vi "Delete by Name.vi"(8 "error in (no error)":errorcluster, 11 "buffer_name":string="/example") -> (0 "error out":errorcluster)   [LabVIEW 2021, in "CIF_NI_CIPC.lvlib"]
doc: "Removes a CIPC buffer from the system."
uses:
  CIF_NI_CIPC.lvlib
  libnicipc.dll
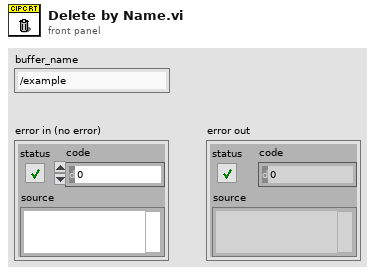
[diagram p1: front panel]
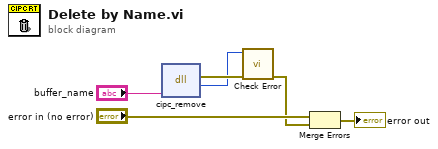
[diagram p0: block diagram]
diagram:
  n1 = dll-call lib="libnicipc.*" fn="cipc_remove"("name"="buffer_name") -> (error out=w6:errorcluster, "return type"=w5:i32)  [unwired: 4 in, 1 out]
  n2 = call "Check Error.vi"("error in (no error)"=w6, "Error Code"=w5) -> ("error out"=w2:errorcluster)  [unwired: 9 in]
  n3 = Merge Errors("error in (no error)", w2) -> (→"error out":errorcluster)
